vi "Frequency Spectrum.vi"() -> ()   [LabVIEW 2010]
uses:
  <vilib>/DAQmx/read.llb/DAQmx Read (Analog Wfm 1Chan NSamp).vi
  <vilib>/DAQmx/create/channels.llb/DAQmx Create Channel (AI-Voltage-Basic).vi
  <vilib>/DAQmx/configure/timing.llb/DAQmx Timing (Sample Clock).vi
  <vilib>/Analysis/2dsp.llb/Real FFT.vi
  <vilib>/measure/maspectr.llb/FFT Spectrum (Mag-Phase) for 1 Chan.vi
  <vilib>/daqmx/miscellaneous.llb/DAQmx Fill In Error Info.vi
  <vilib>/measure/NI_MAPro.lvlib
  <vilib>/Analysis/NI_AALPro.lvlib
panel:
  out "Waveform Graph":waveform(dbl)(graph)
  out "Time Domain Graph":waveform(dbl)(graph)
  in  "physical channels":tag
  in  "window":T1(ring)
  out "Waveform Spectrum":cluster{"f0":dbl, "df":dbl, "magnitude":dbl[]}(graph)
  in  "Stop":bool
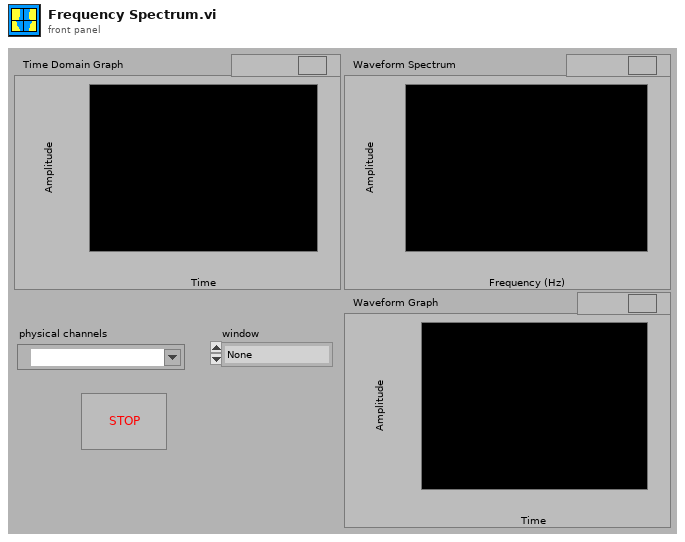
[diagram p1: front panel]
types:
  T1 = enum16{"None ", "Hanning", "Hamming", "Blackman-Harris", "Exact Blackman", "Blackman", "Flat Top", "4 Term B-Harris ", "7 Term B-Harris", "Low Sidelobe"}
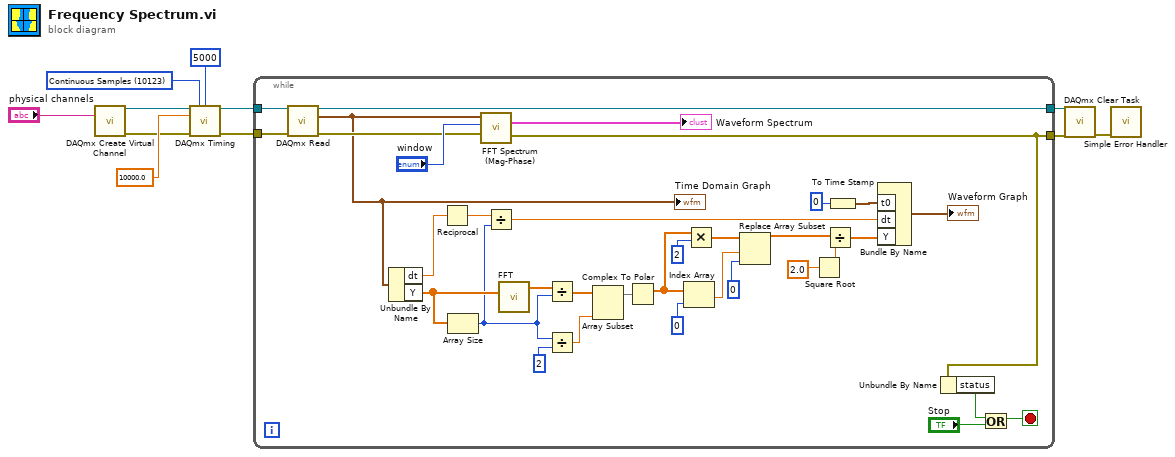
[diagram p0: block diagram]
diagram:
  w9 = 10123 items=["Finite Samples"=10178, "Continuous Samples"=10123] ("sample mode")
  n1 = call-poly <vilib>:"DAQmx Create Virtual Channel.vi"("physical channels"="physical channels") -> ("task out"=w6:refnum<k21>, "error out"=w5:errorcluster)  [unwired: 13 in]
  n2 = call-poly <vilib>:"DAQmx Timing.vi"("task/channels in"=w6, "sample mode"=w9, "samples per channel"=5000, "rate"=10000.0, "error in"=w5) -> ("task out"=w3:refnum<k21>, "error out"=w2:errorcluster)  [unwired: 9 in]
  n3 = while {
    tunnel: [w25] -> w4
    tunnel: w3 -> [w17]
    tunnel: w2 -> [w16]
    tunnel: [w14] -> w1
    stop <- w23 stop-if-true
    n4 = call-poly <vilib>:"DAQmx Read.vi"("task/channels in"=w17, "error in"=w16) -> ("task out"=w14:refnum<k21>, "data"=w12:waveform(dbl), "error out"=w15:errorcluster)  [unwired: 11 in]
    "Time Domain Graph" <- w12
    n5 = Unbundle By Name ("Get Waveform Components")(w12) -> ("dt"=w43:dbl, "Y"=w42:dbl[])
    n6 = Reciprocal(x=w43) -> (1/x=w41:dbl)
    n7 = Array Size(array=w42) -> (size(s)=w37:i32)
    n8 = call-poly <vilib>:"FFT Spectrum (Mag-Phase).vi"("error in (no error)"=w15, "window"="window", "time signal"=w12) -> ("error out"=w25:errorcluster, "magnitude"=→"Waveform Spectrum":cluster{"f0":dbl, "df":dbl, "magnitude":dbl[]})  [unwired: 4 in, 3 out]
    n9 = Divide(x=w41, y=w37) -> (x/y=w38:dbl)
    n10 = call-poly <vilib>:"FFT.vi"("X"=w42) -> ("FFT {X}"=w40:cdb[])  [unwired: 9 in, 1 out]
    n11 = Divide(x=w40, y=w37) -> (x/y=w35:cdb[])
    n12 = Divide(x=w37, y=2) -> (x/y=w34:dbl)
    n13 = Array Subset "Array Subset"(array=w35, length=w34) -> (w33:cdb[])  [unwired: 1 in]
    n14 = Complex To Polar(r * e^(i*theta)=w33) -> (r=w31:dbl[])  [unwired: 1 out]
    n15 = Index Array "Index Array"(array=w31, index=0) -> (element=w28:dbl)
    n16 = Multiply(x=w31, y=2) -> (x*y=w29:dbl[])
    n17 = Replace Array Subset(array=w29, new element=0, index=w28) -> (w20:dbl[])
    n18 = Square Root(x=2.0) -> (sqrt(x)=w21:dbl)
    n19 = Divide(x=w20, y=w21) -> (x/y=w19:dbl[])
    n20 = To Time Stamp(1:0) -> (0:w18:timestamp)
    n21 = Bundle By Name ("Build Waveform")("t0"=w18, "dt"=w38, "Y"=w19) -> (→"Waveform Graph":waveform(dbl))  [unwired: 1 in]
    n22 = Unbundle By Name(w25) -> ("status"=w24:bool)
    n23 = Or(x=w24, y="Stop") -> (x .or. y?=w23:bool)
  }
  n24 = call <vilib>:"DAQmx Clear Task.vi"("task in"=w1, "error in"=w4) -> ("error out"=w11:errorcluster)  [unwired: 13 in]
  n25 = call <vilib>:"Simple Error Handler.vi"("error in (no error)"=w11) -> ()  [unwired: 4 in, 5 out]
